vi "Chemyx_Syringe_Pump_BasicExample.vi"() -> ()   [LabVIEW 2016]
doc: "The basic example uses a general design pattern based on a while loop and an event structure to demonstrate basic operations of the LabVIEW driver for Chemyx syringe pumps.\nCommunication settings (Port and Baud rate) must be set before running this VI.\nThe basic example can be used to start, stop, and pause operations of the syringe pumps. The pump must be manually configured directly on the pump.\nThe status of the pump is queried and displayed."
uses:
  _driver/Basic driver/Status/controls/Pump_status_enum.ctl
  _driver/Basic driver/Communication/controls/comm_rate_enum.ctl
  _driver/_private/Control/Control Mode.ctl
  _driver/_private/Control/Programmable Mode.ctl
  _driver/Chemyx_Syringe_Pump_driver.lvlib
panel:
  in  "Mode":T1=enum."Basic"
  in  "[x]":T2
  out "Connection":bool
  out "Limits":dbl[](array[numeric])
  in  "Baud rate":T3
  out "Status":T4
  in  "Quit Button":bool
  in  "Port":refnum<visa-resource-name>
  out "Dispensed volume":dbl
  out "Elapsed time":string
  in  "Reset Button":bool
  in  "Pause Button":bool
  in  "Stop Button":bool
  in  "Start Button":bool
  # "Communication Settings"
  # "Commands"
  # "Status"
  # "Select Port and Baud rate before running the VI.\n\nSimple VI demonstrating the use of the Basic driver to control a Chemyx syringe pump."
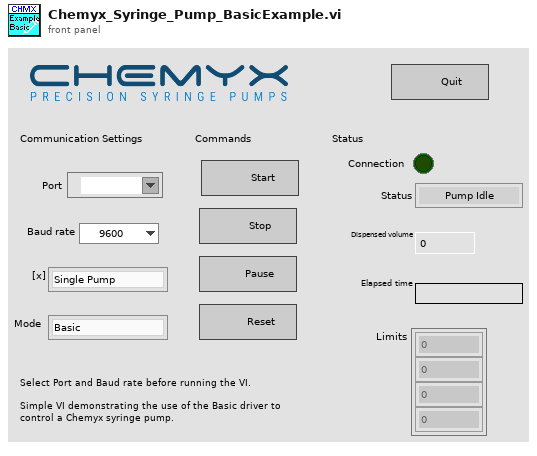
[diagram p1: front panel]
types:
  T1 = typedef "Chemyx_Syringe_Pump_driver.lvlib/Programmable Mode.ctl" = enum16{"Blank", "Basic", "Programmable"}
  T2 = typedef "Chemyx_Syringe_Pump_driver.lvlib/Control Mode.ctl" = enum16{"Single Pump", "Pump Channel 1", "Pump Channel 2", "Cycle Mode"}
  T3 = typedef "Chemyx_Syringe_Pump_driver.lvlib/comm_rate_enum.ctl" = enum16{"9600", "38400"}
  T4 = typedef "Chemyx_Syringe_Pump_driver.lvlib/Pump_status_enum.ctl" = enum16{"Pump Idle", "Pump Running", "Pump Paused", "Pump Delay", "Pump Stalled", "Pump Error"}
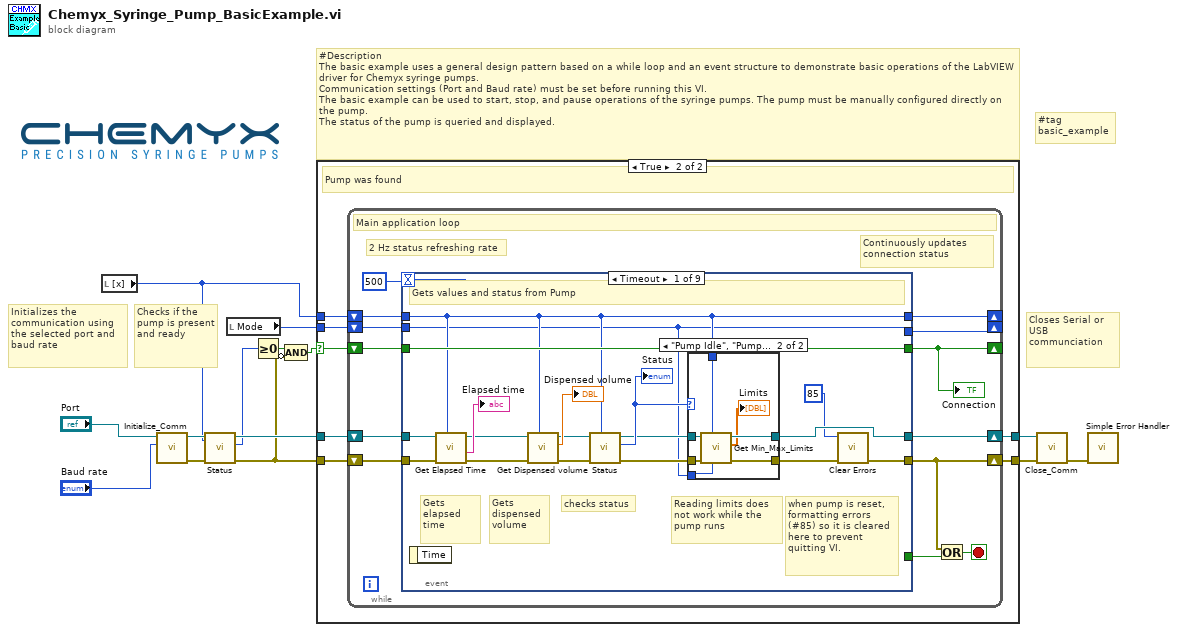
[diagram p0: block diagram]
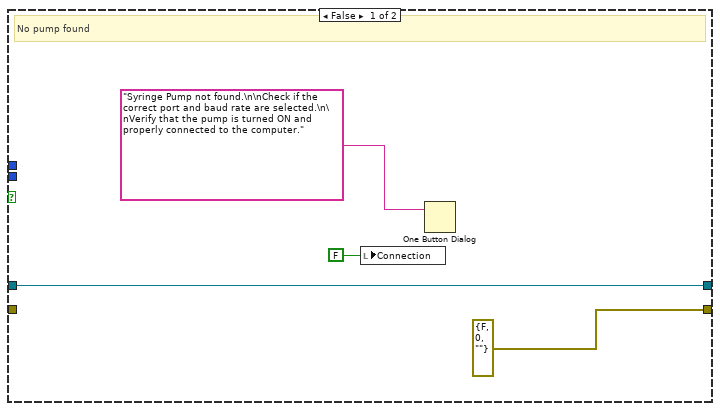
[diagram p2: hidden frame]
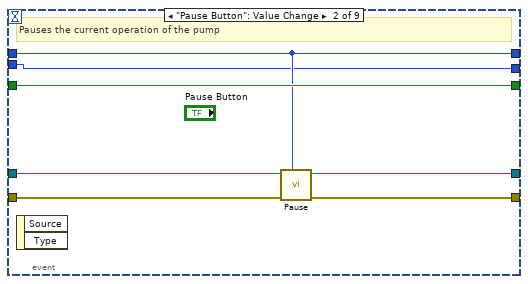
[diagram p4: hidden frame]
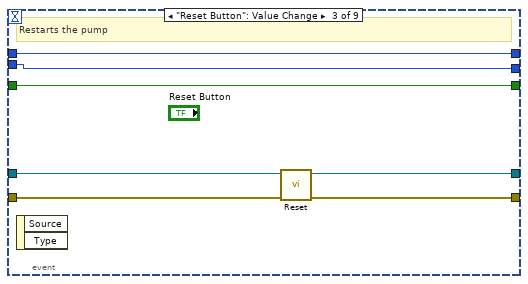
[diagram p5: hidden frame]
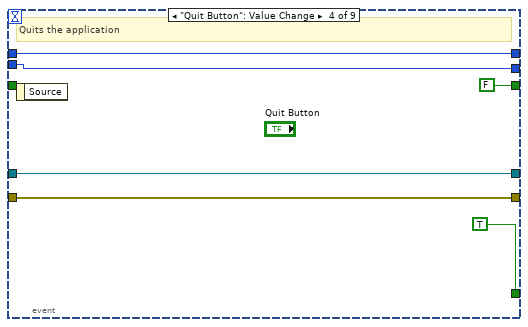
[diagram p6: hidden frame]
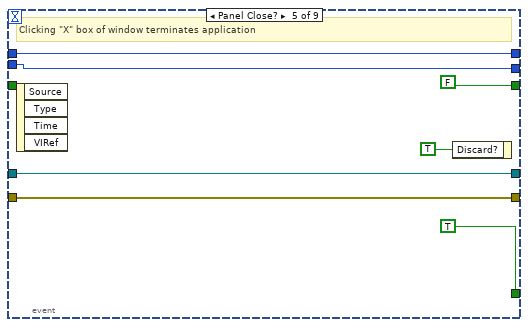
[diagram p7: hidden frame]
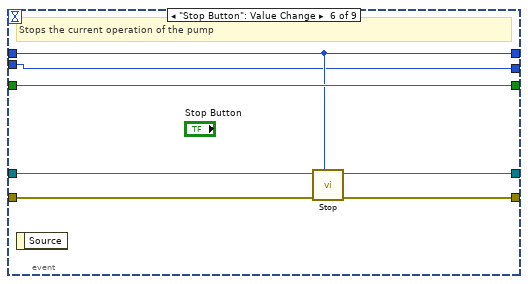
[diagram p8: hidden frame]
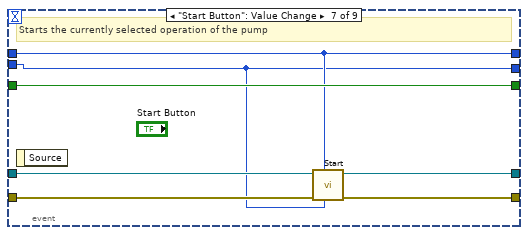
[diagram p9: hidden frame]
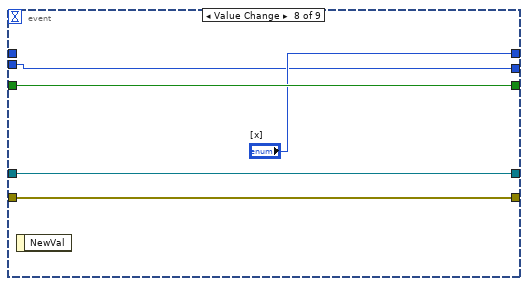
[diagram p10: hidden frame]
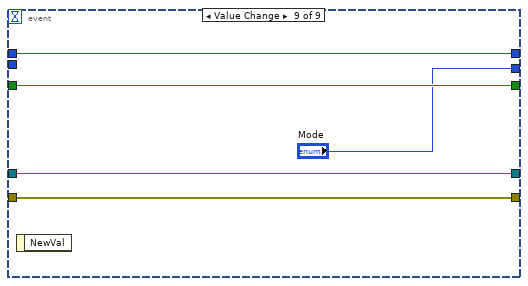
[diagram p11: hidden frame]
diagram:
  # "#tag\nbasic_example"
  # "#Description\nThe basic example uses a general design pattern based on a while loop and an event structure to demonstrate basic operations of the LabVIEW driver for Chemyx syringe pumps.\nCommunication settings (Port and Baud rate) must be set before running this VI.\nThe basic example can be used to start, stop, and pause operations of the syringe pumps. The pump must be manually configured directly on the pump.\nThe status of the pump is queried and displayed."
  # "Closes Serial or USB communciation"
  # "Checks if the pump is present and ready"
  # "Initializes the communication using the selected port and baud rate"
  n1 = local read "[x]"() -> (w2:T2)
  n2 = call "Initialize_Comm.vi"("Baud rate"="Baud rate", "Serial Port in"="Port") -> ("error out"=w13:errorcluster, "Serial Port out"=w8:refnum<visa-resource-name>)  [unwired: 8 in]
  n3 = call "Status.vi"("[x]"=w2, "error in (no error)"=w13, "Serial Port in"=w8) -> ("error out"=w3:errorcluster, "Status"=w6:T4, "Serial Port out"=w7:refnum<visa-resource-name>)  [unwired: 6 in]
  n4 = local read "Mode"() -> (w1:T1)
  n5 = Greater Or Equal To 0?(x=w6) -> (x >= 0?=w5:bool)
  n6 = Compound Arithmetic op=AND(w5, invert w3) -> (w4:bool)
  n7 = case shown="True" w4 {
    selector: w4 -> [_ w21]
    tunnel: [errorcluster {"status"=FALSE, "code"=0, "source"=""} ("error out") w25] -> w11
    tunnel: [w18 w24] -> w9
    tunnel: w3 -> [_ w23]
    tunnel: w7 -> [w18 w22]
    tunnel: w2 -> [_ w20]
    tunnel: w1 -> [_ w19]
    frame False {
      # "No pump found"
      n8 = local write "Connection"(FALSE ("Connection")) -> ()
      n9 = One Button Dialog(message="Syringe Pump not found.\n\nCheck if the correct port and baud rate are selected.\n\nVerify that the pump is turned ON and properly connected to the computer.") -> ()  [unwired: 1 in, 1 out]
    }
    frame True {
      # "Pump was found"
      n10 = while {
        shift-right: [w33] -> w25
        shift-left: w23 -> [w37]
        shift-right: [w32] -> w24
        shift-left: w22 -> [w36]
        shift-right: [w30] -> _
        shift-left: w21 -> [w31]
        shift-right: [w28] -> _
        shift-left: w20 -> [w29]
        shift-right: [w27] -> _
        shift-left: w19 -> [w26]
        stop <- w34 stop-if-true
        # "2 Hz status refreshing rate"
        # "Continuously updates connection status"
        # "Main application loop"
        n11 = event shown="[0] Timeout" {
          selector: _ -> [_ _ _ _ _ _ _ _ _]
          dyn-events: _ -> [_ _ _ _ _ _ _ _ _]
          timeout: 500 -> [_ _ _ _ _ _ _ _ _]
          tunnel: [_ _ _ TRUE TRUE _ _ _ _] -> w38
          tunnel: w37 -> [w46 w68 w75 w82 w89 w96 w105 w106 w111]
          tunnel: [w42 w71 w78 w82 w89 w98 w104 w106 w111] -> w33
          tunnel: w36 -> [w45 w69 w76 w83 w90 w95 w103 w107 w112]
          tunnel: [w49 w70 w77 w83 w90 w97 w102 w107 w112] -> w32
          tunnel: w31 -> [w48 w67 w74 _ _ w94 w101 w110 w115]
          tunnel: [w48 w67 w74 FALSE FALSE w94 w101 w110 w115] -> w30
          tunnel: w29 -> [w40 w66 w73 w80 w86 w93 w100 _ w114]
          tunnel: [w40 w66 w73 w80 w86 w93 w100 "[x]" w114] -> w28
          tunnel: [w39 w65 w72 w79 w85 w92 w99 w108 "Mode"] -> w27
          tunnel: w26 -> [w39 w65 w72 w79 w85 w92 w99 w108 _]
          event Timeout {
            # "when pump is reset, formatting errors (#85) so it is cleared here to prevent quitting VI."
            # "Gets dispensed volume"
            # "Gets elapsed time"
            # "checks status"
            # "Reading limits does not work while the pump runs"
            # "Gets values and status from Pump"
            n12 = event-data() -> ()  [unwired: 1 in, 1 out]
            n13 = call "Get Elapsed Time.vi"("[x]"=w40, "error in (no error)"=w46, "Serial Port in"=w45) -> ("error out"=w55:errorcluster, "Time string"=→"Elapsed time":string, "Serial Port out"=w52:refnum<visa-resource-name>)  [unwired: 6 in]
            n14 = call "Get Dispensed volume.vi"("[x]"=w40, "error in (no error)"=w55, "Serial Port in"=w52) -> ("error out"=w53:errorcluster, "Volume"=→"Dispensed volume":dbl, "Serial Port out"=w43:refnum<visa-resource-name>)  [unwired: 6 in]
            n15 = call "Status.vi"("[x]"=w40, "Serial Port in"=w43) -> ("Status"=w47:T4, "Serial Port out"=w44:refnum<visa-resource-name>)  [unwired: 7 in, 1 out]
            "Status" <- w47
            n16 = case shown="\"Pump Idle\", \"Pump Paused\", \"Pump Delay\"" w47 {
              tunnel: w53 -> [w56 w64]
              tunnel: [w56 w63] -> w50
              tunnel: w44 -> [w57 w62]
              tunnel: [w57 w61] -> w49
              tunnel: w40 -> [_ w59]
              tunnel: w39 -> [_ w58]
              frame "Pump Running", Default {
              }
              frame "Pump Idle", "Pump Paused", "Pump Delay" {
                n17 = call "Get Min_Max_Limits.vi"("Mode"=w58, "[x]"=w59, "error in (no error)"=w64, "Serial Port in"=w62) -> ("error out"=w63:errorcluster, "Limits"=→"Limits":dbl[], "Serial Port out"=w61:refnum<visa-resource-name>)  [unwired: 5 in]
              }
            }
            n18 = call <vilib>:"Clear Errors.vi"("error in (no error)"=w50, "specific error code to clear (0: all)"=85) -> ("error out"=w42:errorcluster)  [unwired: 4 in, 1 out]
          }
          event "Pause Button": Value Change {
            # "Pauses the current operation of the pump"
            n19 = event-data() -> ()  [unwired: 1 in, 2 out]
            n20 = call "Pause.vi"("[x]"=w66, "error in (no error)"=w68, "Serial Port in"=w69) -> ("error out"=w71:errorcluster, "Serial Port out"=w70:refnum<visa-resource-name>)  [unwired: 7 in]
          }
          event "Reset Button": Value Change {
            # "Restarts the pump"
            n21 = event-data() -> ()  [unwired: 1 in, 2 out]
            n22 = call "Reset.vi"("error in (no error)"=w75, "Serial Port in"=w76) -> ("error out"=w78:errorcluster, "Serial Port out"=w77:refnum<visa-resource-name>)  [unwired: 8 in]
          }
          event "Quit Button": Value Change {
            # "Quits the application"
            n23 = event-data() -> ()  [unwired: 1 in, 1 out]
          }
          event Panel Close? {
            # "Clicking \"X\" box of window terminates application"
            n24 = event-data() -> ()  [unwired: 1 in, 4 out]
            n25 = event-data("Discard?"=TRUE) -> ()  [unwired: 1 in, 1 out]
          }
          event "Stop Button": Value Change {
            # "Stops the current operation of the pump"
            n26 = event-data() -> ()  [unwired: 1 in, 1 out]
            n27 = call "Stop.vi"("[x]"=w93, "error in (no error)"=w96, "Serial Port in"=w95) -> ("error out"=w98:errorcluster, "Serial Port out"=w97:refnum<visa-resource-name>)  [unwired: 7 in]
          }
          event "Start Button": Value Change {
            # "Starts the currently selected operation of the pump"
            n28 = event-data() -> ()  [unwired: 1 in, 1 out]
            n29 = call "Start.vi"("Mode"=w99, "[x]"=w100, "error in (no error)"=w105, "Serial Port in"=w103) -> ("error out"=w104:errorcluster, "Serial Port out"=w102:refnum<visa-resource-name>)  [unwired: 6 in]
          }
          event Value Change {
            n30 = event-data() -> ()  [unwired: 1 in, 1 out]
          }
          event Value Change {
            n31 = event-data() -> ()  [unwired: 1 in, 1 out]
          }
        }
        "Connection" <- w30
        n32 = Or(x=w33, y=w38) -> (x .or. y?=w34:bool)
      }
    }
  }
  n33 = call "Close_Comm.vi"("error in (no error)"=w11, "Serial Port in"=w9) -> ("error out"=w10:errorcluster)  [unwired: 9 in]
  n34 = call <vilib>:"Simple Error Handler.vi"("error in (no error)"=w10) -> ()  [unwired: 4 in, 5 out]
